vi "Destructor.vi"(0 "Core In":refnum<class "Core.lvclass">, 11 "Error In":errorcluster {"code" format="%.0x"}) -> (4 "Core Out":refnum<class "Core.lvclass">, 15 "Error Out":errorcluster {"Code" format="%.0x"})   [LabVIEW 2020, in "Core.lvlib" / "Core.lvclass"]
doc: "Destructor of this instance, clears and release any memory usage of the object."
uses:
  Core.lvclass
  DataReference.ctl
  Data.ctl
  Build.ctl
  Core.lvclass/Core.ctl
panel:
  # "/* Inputs */"
  # "/* Locals */"
  # "/* Outputs */"
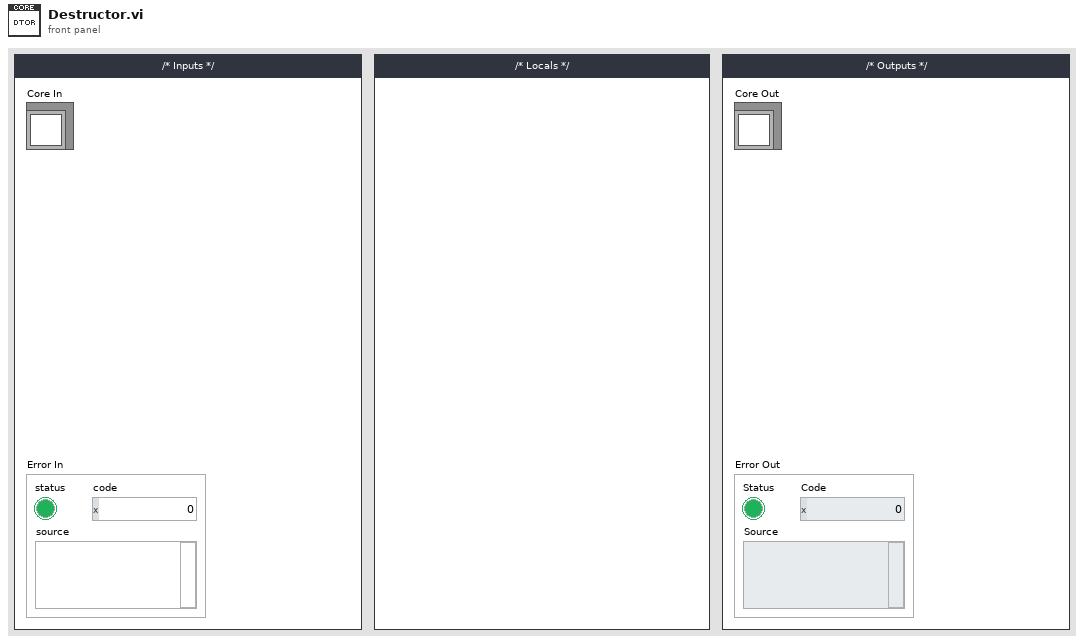
[diagram p1: front panel]
types:
  T1 = typedef "Core.lvlib/Core.lvclass/DataReference.ctl" = refnum<data-value>
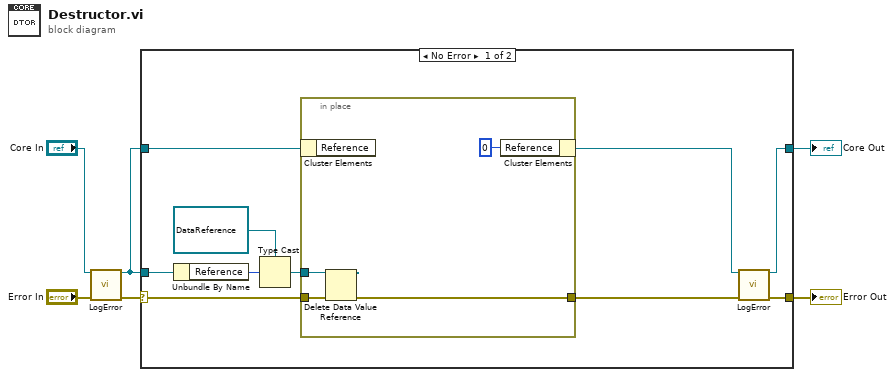
[diagram p0: block diagram]
diagram:
  n1 = call-dynamic "LogError.vi"("Core In"="Core In", "Error In"="Error In") -> ("Core Out"=w1:refnum<class "Core.lvclass">, "Error Out"=w3:errorcluster)  [unwired: 12 in]
  n2 = case shown="No Error" w3 {
    selector: w3 -> [w8 w21]
    tunnel: [w15 w21] -> w6
    tunnel: w1 -> [w10 w22]
    tunnel: [w13 w22] -> w5
    tunnel: w1 -> [w7 _]
    frame No Error {
      n3 = Unbundle By Name(w7) -> ("Reference"=w11:u64)
      n4 = Type Cast(type=T1 refnum ("Data Reference"), x=w11) -> (*(type *) &x=w9:T1)
      n5 = in-place {
        in-place-border: w8 -> [w20]
        in-place-border: [w19] -> w16
        in-place-border: w9 -> [w17]
        n6 = in-place-cluster #1(w10) -> ()  [unwired: 1 out]
        n7 = Delete Data Value Reference(data value reference=w17, error in=w20) -> (error out=w19:errorcluster)  [unwired: 1 out]
        n8 = in-place-cluster #1("Reference"=u64 0) -> (w14:refnum<class "Core.lvclass">)
      }
      n9 = call-dynamic "LogError.vi"("Core In"=w14, "Error In"=w16) -> ("Core Out"=w13:refnum<class "Core.lvclass">, "Error Out"=w15:errorcluster)  [unwired: 12 in]
    }
    frame Error {
    }
  }
  "Core Out" <- w5
  "Error Out" <- w6
